vi "EEI EXP Trial1.vi"() -> ()   [LabVIEW 2020]
panel:
  out "Celcuis 2":dbl
  in  "Fahrenheit 2":dbl
  out "Fahrenheit 1":dbl
  in  "Celcius 1":dbl
  out "current time":timestamp
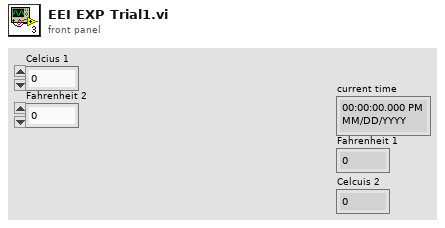
[diagram p1: front panel]
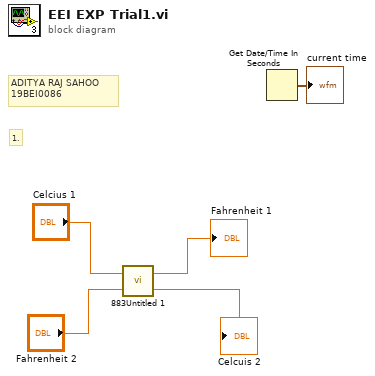
[diagram p0: block diagram]
diagram:
  # "1."
  # "ADITYA RAJ SAHOO\n19BEI0086"
  n1 = call "883Untitled 1.vi"("Fahrenheit 2"="Fahrenheit 2", "Celcius 1"="Celcius 1") -> ("Celcuis 2"=→"Celcuis 2":dbl, "Fahrenheit 1"=→"Fahrenheit 1":dbl)
  n2 = Get Date/Time In Seconds() -> (seconds since 1Jan1904=→"current time":timestamp)
